vi "getFPGA.vi"(11 "ModbusTriggerControl in":refnum<class "ModbusTriggerControl.lvclass">) -> (2 "FPGA":refnum<class "FPGA.lvclass">, 3 "ModbusTriggerControl out":refnum<class "ModbusTriggerControl.lvclass">)   [LabVIEW 2016, in "ModbusTriggerControl.lvclass"]
uses:
  ModbusTriggerControl.lvclass
  FPGA/FPGA.lvclass
  ModbusTriggerControl.lvclass/ModbusTriggerControl.ctl
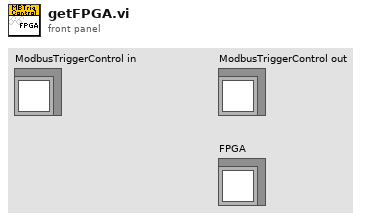
[diagram p1: front panel]
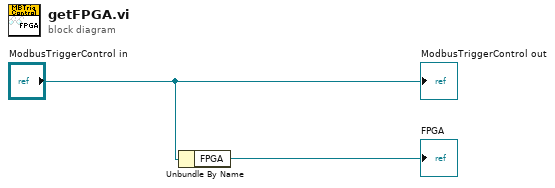
[diagram p0: block diagram]
diagram:
  n1 = Unbundle By Name("ModbusTriggerControl in") -> ("FPGA"=→"FPGA":refnum<class "FPGA.lvclass">)
  "ModbusTriggerControl out" <- "ModbusTriggerControl in"
